vi "IsNewHeaders_True.vi"(8 "error in":errorcluster, 10 "Headers":string[](array[string])=["Numeric Data", "Float Data", "String Data", "Enum Data", "Array Data[0].Numeric Data", "Array Data 2[0].Numeric Data", "Array Data 2[1].Numeric Data"], 11 "Data":string) -> (0 "error out":errorcluster, 2 "Different Header?":bool, 3 "Old Headers":string[](array[string]))   [LabVIEW 2014, in "TableLogger_CSV_Actor.lvlib" / "TableLogger_CSV_Actor.lvclass"]
uses:
  TableLogger_CSV_Actor.lvclass
panel:
  # "Connector Pane"
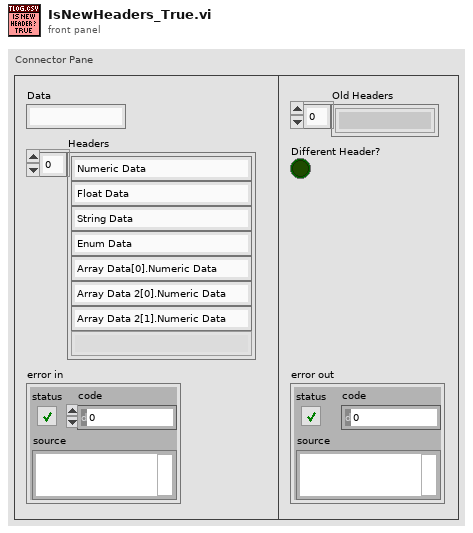
[diagram p1: front panel]
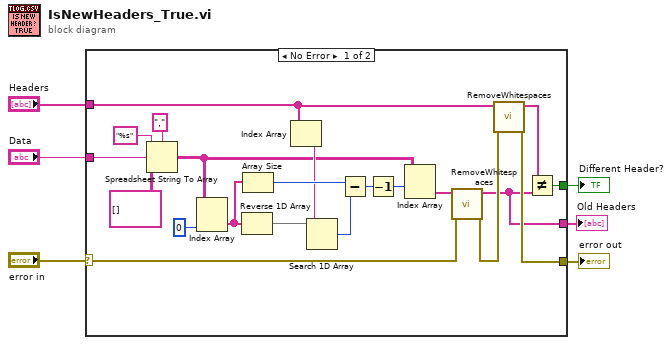
[diagram p0: block diagram]
diagram:
  n1 = case shown="No Error" "error in" {
    selector: "error in" -> [w11 w28]
    tunnel: "Headers" -> [w26 _]
    tunnel: [w24 w28] -> w5
    tunnel: [w23 _] -> w4
    tunnel: "Data" -> [w10 _]
    tunnel: [w7 _] -> w1
    frame No Error {
      n2 = Spreadsheet String To Array(delimiter (Tab)=",", format string="%s", spreadsheet string=w10, array type (2D Dbl)=string[][] []) -> (array=w8:string[][])
      n3 = Index Array(array=w8, index (col)=0 ("disabled index (col)")) -> (element=w17:string[])  [unwired: 1 in]
      n4 = Reverse 1D Array(array=w17) -> (reversed array=w18:string[])
      n5 = Array Size(array=w17) -> (size(s)=w16:i32)
      n6 = Index Array(array=w26) -> (element=w15:string)  [unwired: 1 in]
      n7 = Search 1D Array(1D array=w18, element=w15) -> (index of element=w14:i32)  [unwired: 1 in]
      n8 = Subtract(x=w16, y=w14) -> (x-y=w13:i32)
      n9 = Decrement(x=w13) -> (x-1=w12:i32)
      n10 = Index Array(array=w8, index (row)=w12) -> (element=w27:string[])  [unwired: 1 in]
      n11 = call "RemoveWhitespaces.vi"("error in (no error)"=w11, "Array In"=w27) -> ("error out"=w25:errorcluster, "Array removing empty space"=w7:string[])  [unwired: 8 in]
      n12 = call "RemoveWhitespaces.vi"("error in (no error)"=w25, "Array In"=w26) -> ("error out"=w24:errorcluster, "Array removing empty space"=w9:string[])  [unwired: 8 in]
      n13 = Not Equal?(x=w9, y=w7) -> (x != y?=w23:bool)
    }
    frame Error {
    }
  }
  "error out" <- w5
  "Different Header?" <- w4
  "Old Headers" <- w1
